vi "FRCts20_Backend_Test_Event_PUT.vi"(8 "error in (no error)":errorcluster, 11 "Event Out":T1) -> (0 "error out":errorcluster, 1 "Time (ms)":u32, 2 "Status":string, 3 "Event Out":T1, 5 "Success":bool)   [LabVIEW 2013, in "FRCts20_Backend_TestCode.lvlib"]
uses:
  FRCts20_Backend_TestCode.lvlib
  FRCts20_Backend_API/FRCts20_Backend_API_Event.ctl
  FRCts20_Backend_API/FRCts20_Backend_API_SW.ctl
  FRCts20_Backend_API/FRCts20_Backend_API_Command_Event.ctl
  FRCts20_Backend_API/FRCts20_Backend_API_Event.vi
  FRCts20_Backend_API/FRCts20_Backend_API.lvlib
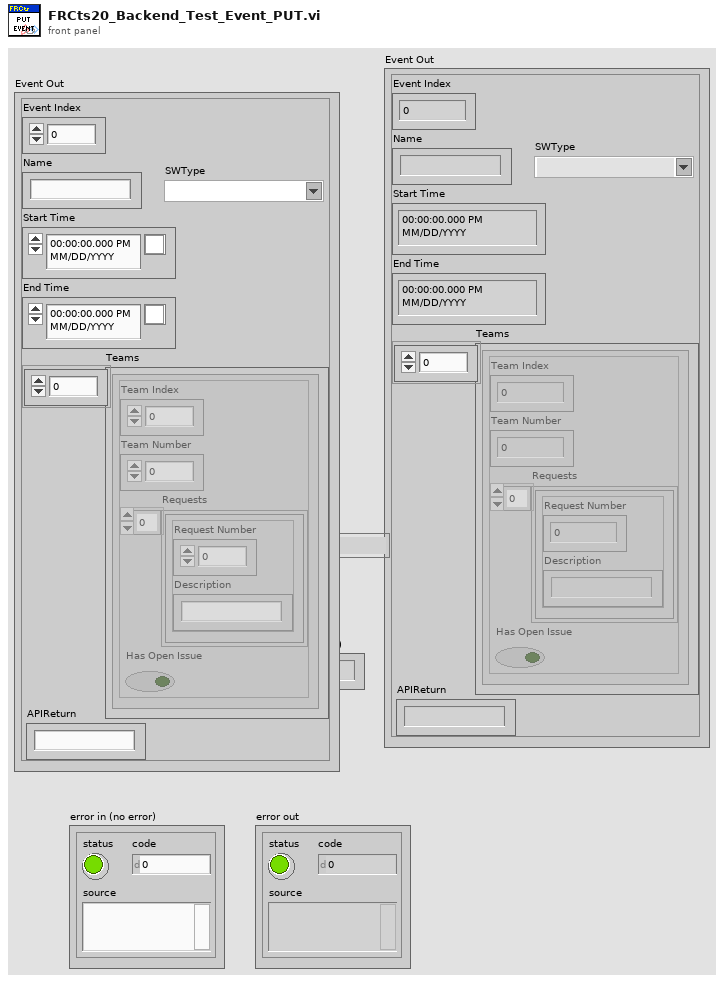
[diagram p1: front panel]
types:
  T1 = typedef "FRCts20_Backend_API.lvlib/FRCts20_Backend_API_Event.ctl" = cluster{"Event Index":u32, "Name":string, "Start Time":timestamp, "End Time":timestamp, "Teams":cluster{"Team Index":u32, "Team Number":u32, "Requests":cluster{"Request Number":u32, "Description":string}[], "Has Open Issue":bool}[], "SWType":T2, "APIReturn":string}
  T2 = typedef "FRCts20_Backend_API.lvlib/FRCts20_Backend_API_SW.ctl" = string
  T3 = typedef "FRCts20_Backend_API.lvlib/FRCts20_Backend_API_Command_Event.ctl" = string
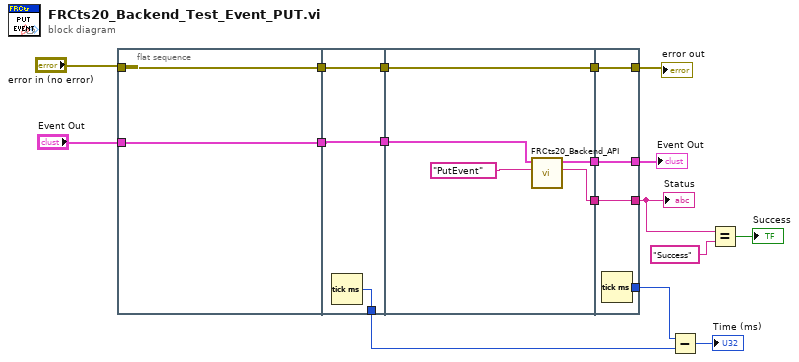
[diagram p0: block diagram]
diagram:
  n1 = flat-sequence {
    tunnel: "error in (no error)" -> [w19]
    tunnel: [w19] -> w17
    tunnel: [w18] -> w2
    tunnel: "Event Out" -> [w18]
    tunnel: [w22] -> w5
    tunnel: [w21] -> w16
    tunnel: w17 -> [w21]
    tunnel: [w20] -> w15
    tunnel: w2 -> [w20]
    tunnel: [w27] -> w14
    tunnel: w16 -> [w27]
    tunnel: w15 -> [w25]
    tunnel: [w24] -> w13
    tunnel: [w23] -> w12
    tunnel: [w31] -> w6
    tunnel: [w30] -> w8
    tunnel: w14 -> [w30]
    tunnel: [w29] -> w4
    tunnel: w13 -> [w29]
    tunnel: [w28] -> w3
    tunnel: w12 -> [w28]
    frame #0 {
    }
    frame #1 {
      n2 = Tick Count (ms)() -> (millisecond timer value=w22:u32)
    }
    frame #2 {
      n3 = call-poly "FRCts20_Backend_API.vi"("Command"=T3 "PutEvent", "Event In"=w25) -> ("Status"=w23:string, "Event Out"=w24:T1)  [unwired: 7 in, 1 out]
    }
    frame #3 {
      n4 = Tick Count (ms)() -> (millisecond timer value=w31:u32)
    }
  }
  n5 = Subtract(x=w6, y=w5) -> (x-y=→"Time (ms)":u32)
  n6 = Equal?(x=w3, y="Success") -> (x = y?=→"Success":bool)
  "Event Out" <- w4
  "Status" <- w3
  "error out" <- w8
